vi "Smoothing.vi"(0 "VISA IN":refnum<visa-resource-name>, 5 "error in":errorcluster, 7 "Channel":i32=1, 9 "Percentage Value":i32, 11 "Measurement":string="InputRL") -> (14 "VISA Out":refnum<visa-resource-name>, 19 "error out":errorcluster)   [LabVIEW 2018, in "PNA-X.lvlib"]
uses:
  PNA-X.lvlib
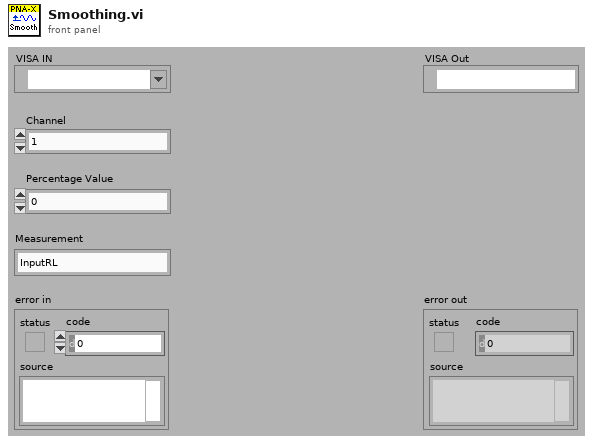
[diagram p1: front panel]
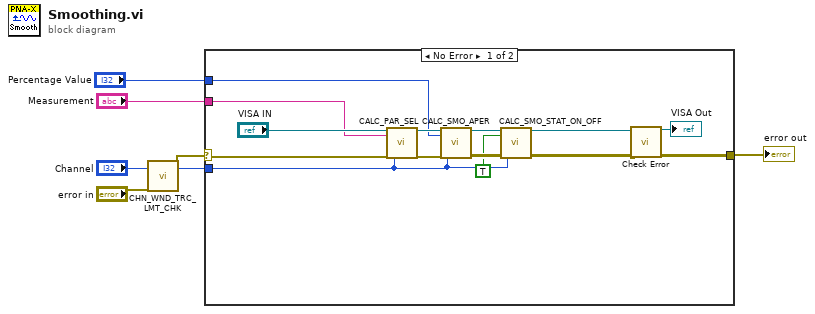
[diagram p0: block diagram]
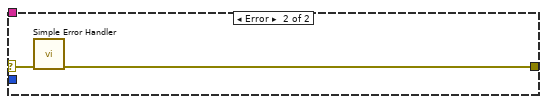
[diagram p2: hidden frame]
diagram:
  n1 = call "CHN_WND_TRC_LMT_CHK.vi"("Channel"="Channel", "error in"="error in") -> ("error out"=w5:errorcluster, "Channel"=w3:i32)  [unwired: 13 in, 3 out]
  n2 = case shown="No Error" w5 {
    selector: w5 -> [w11 w23]
    tunnel: [w21 w22] -> w6
    tunnel: w3 -> [w10 _]
    tunnel: "Measurement" -> [w9 _]
    tunnel: "Percentage Value" -> [w8 _]
    frame No Error {
      n3 = call "CALC_PAR_SEL.vi"("VISA IN"="VISA IN", "Measurement"=w9, "error in"=w11, "Channel"=w10) -> ("VISA Out"=w18:refnum<visa-resource-name>, "error out"=w19:errorcluster)  [unwired: 14 in]
      n4 = call "CALC_SMO_APER.vi"("VISA IN"=w18, "Percentage Value"=w8, "error in"=w19, "Channel"=w10) -> ("VISA Out"=w17:refnum<visa-resource-name>, "error out"=w16:errorcluster)  [unwired: 14 in]
      n5 = call "CALC_SMO_STAT_ON_OFF.vi"("VISA IN"=w17, "Smoothing ON/OFF"=TRUE, "error in"=w16, "Channel"=w10) -> ("VISA Out"=w13:refnum<visa-resource-name>, "error out"=w12:errorcluster)  [unwired: 14 in]
      n6 = call "Check Error.vi"("VISA Resource Name"=w13, "error in (no error)"=w12) -> ("dup VISA session"=→"VISA Out":refnum<visa-resource-name>, "error out"=w21:errorcluster)  [unwired: 16 in]
    }
    frame Error {
      n7 = call <vilib>:"Simple Error Handler.vi"("error in (no error)"=w23) -> ("error out"=w22:errorcluster)  [unwired: 4 in, 4 out]
    }
  }
  "error out" <- w6
